vi "GenServer.vi"(8 "error in":errorcluster, 10 "Default Server":T1, 11 "Server":T1) -> (0 "error out":errorcluster, 2 "Unique Handlers":bool, 3 "Lines":string[](array[string]))   [LabVIEW 2017]
uses:
  <vilib>/WebServerConfig/Server.ctl
  <vilib>/WebServerConfig/Alias.ctl
  <vilib>/WebServerConfig/ErrorDocument.ctl
  <vilib>/WebServerConfig/Action.ctl
  <vilib>/WebServerConfig/Redirect.ctl
  <vilib>/WebServerConfig/Interface.ctl
  <vilib>/WebServerConfig/AddHandler.ctl
  <vilib>/WebServerConfig/SSL.ctl
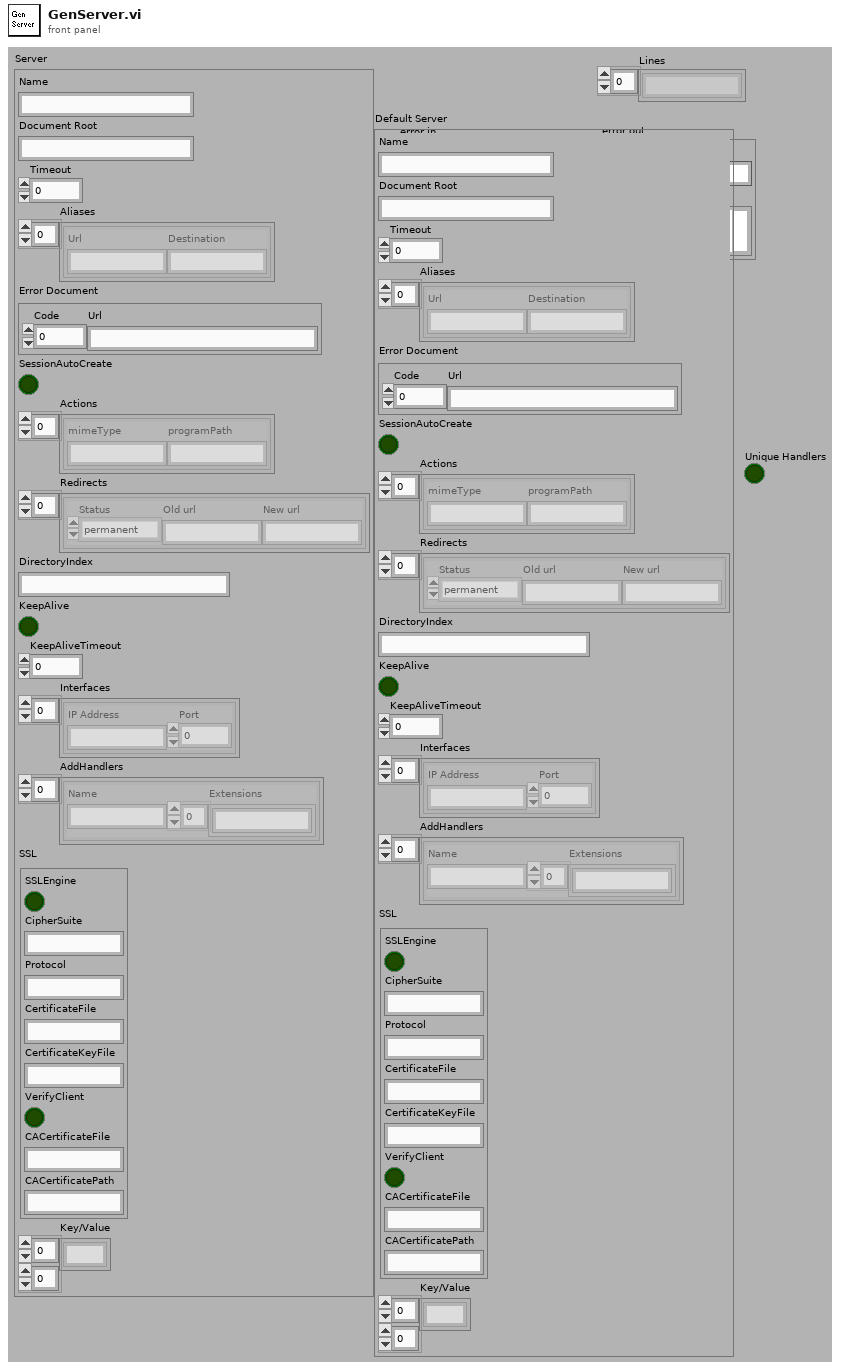
[diagram p1: front panel]
types:
  T1 = typedef "Server.ctl" = cluster{"Name":string, "Document Root":string, "Timeout":u32, "Aliases":T2[], "Error Document":T3, "SessionAutoCreate":bool, "Actions":T4[], "Redirects":T5[], "DirectoryIndex":string, "KeepAlive":bool, "KeepAliveTimeout":u32, "Interfaces":T6[], "AddHandlers":T7[], "SSL":T8, "Key/Value":string[][]}
  T2 = typedef "Alias.ctl" = cluster{"Url":string, "Destination":string}
  T3 = typedef "ErrorDocument.ctl" = cluster{"Code":u16, "Url":string}
  T4 = typedef "Action.ctl" = cluster{"mimeType":string, "programPath":string}
  T5 = typedef "Redirect.ctl" = cluster{"Status":enum16{"permanent", "temp", "seeother", "gone"}, "Old url":string, "New url":string}
  T6 = typedef "Interface.ctl" = cluster{"IP Address":string, "Port":u16}
  T7 = typedef "AddHandler.ctl" = cluster{"Name":string, "Extensions":string[]}
  T8 = typedef "SSL.ctl" = cluster{"SSLEngine":bool, "CipherSuite":string, "Protocol":string, "CertificateFile":string, "CertificateKeyFile":string, "VerifyClient":bool, "CACertificateFile":string, "CACertificatePath":string}
  T9 = enum16{"ServerName", "DocumentRoot", "InactivityTimeout", "AddPipeline", "DirectoryIndex", "Aliases", "ErrorDocument", "SSLEngine", "SSLCertificateFile", "SSLCertificateKeyFile", "SSLVerifyClient", "Key/Value"}
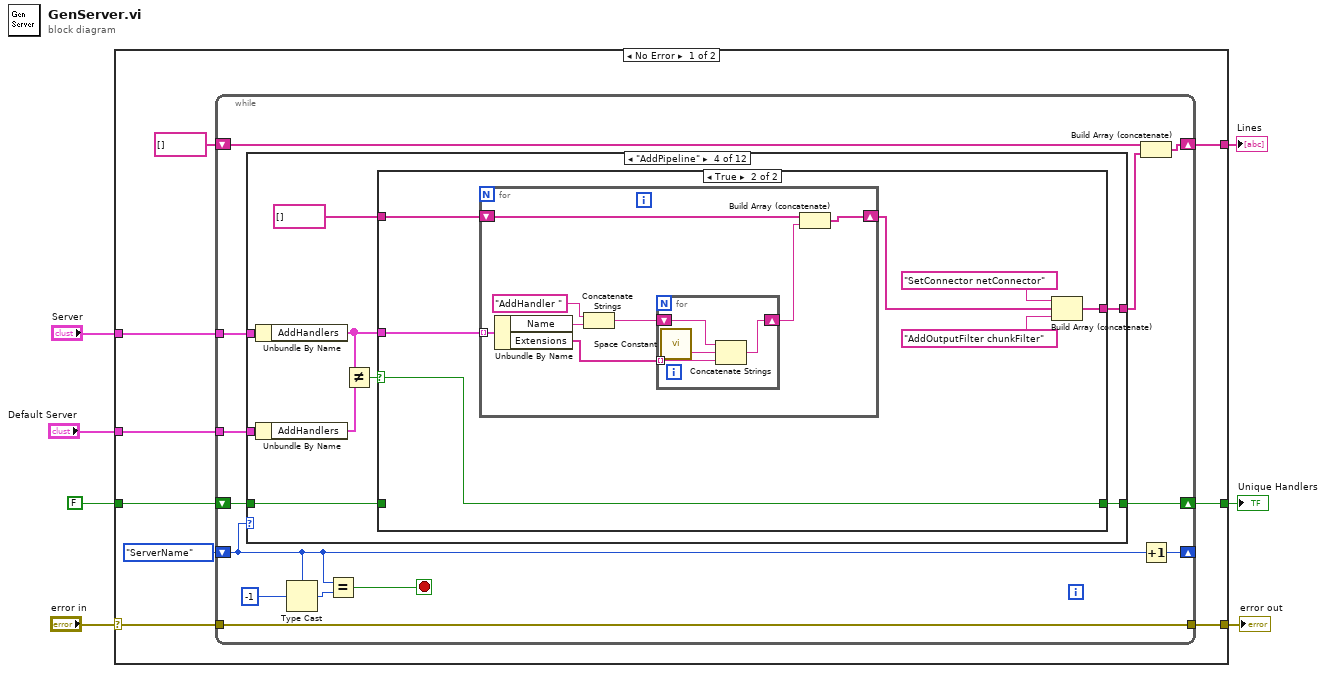
[diagram p0: block diagram]
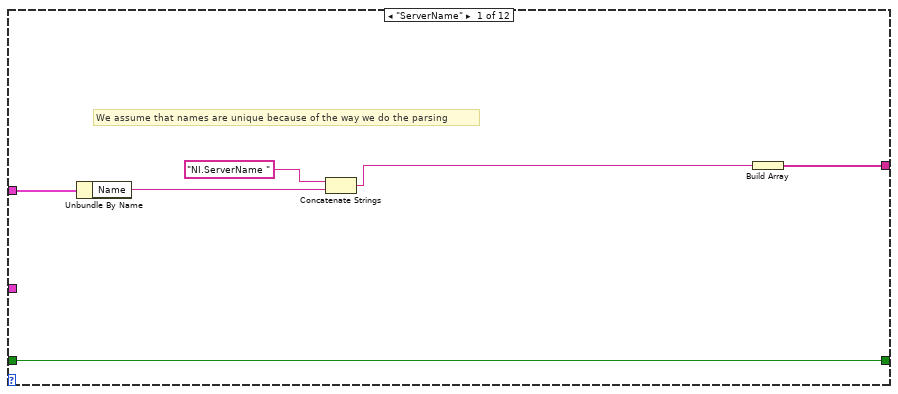
[diagram p2: hidden frame]
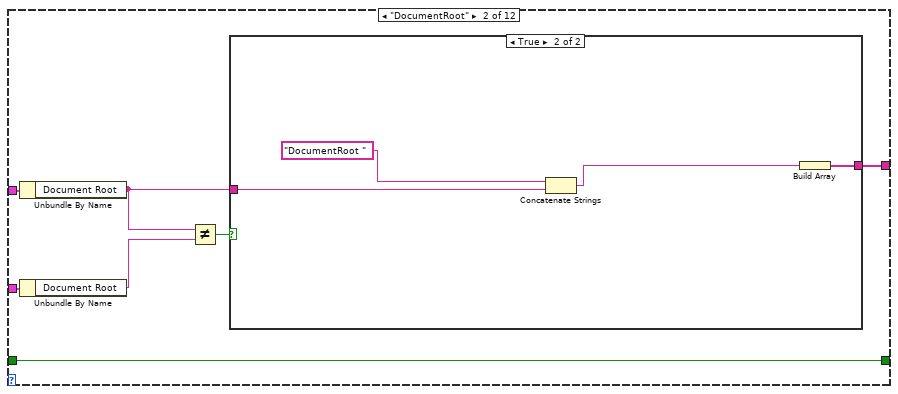
[diagram p3: hidden frame]
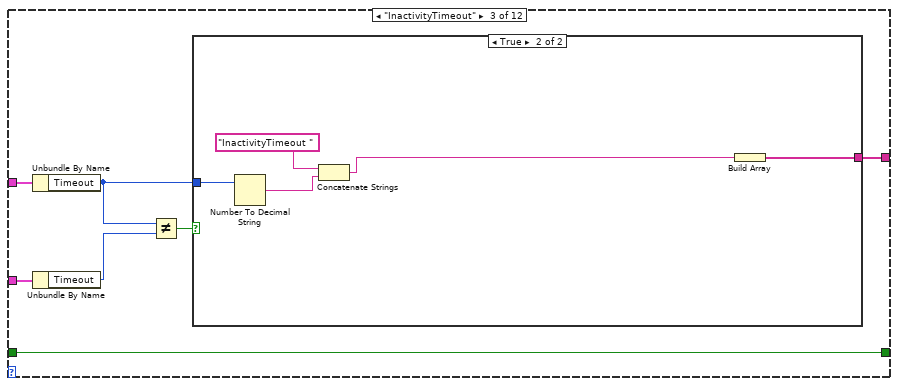
[diagram p5: hidden frame]
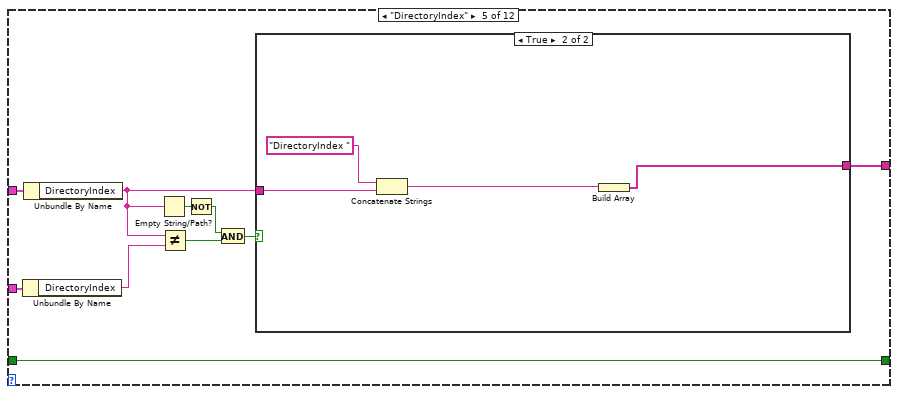
[diagram p8: hidden frame]
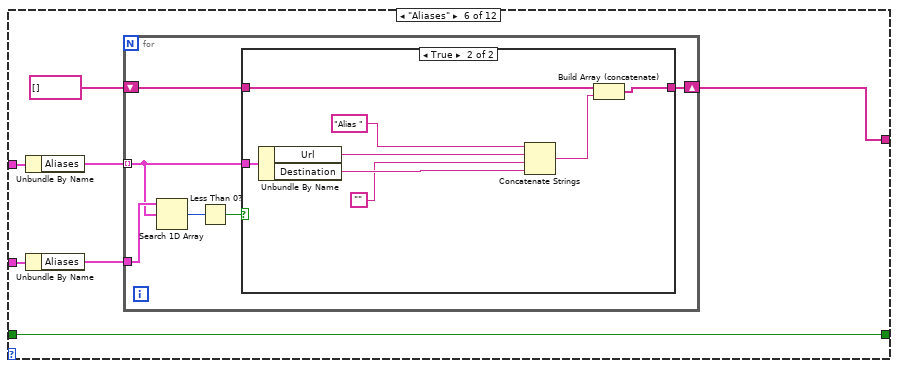
[diagram p10: hidden frame]
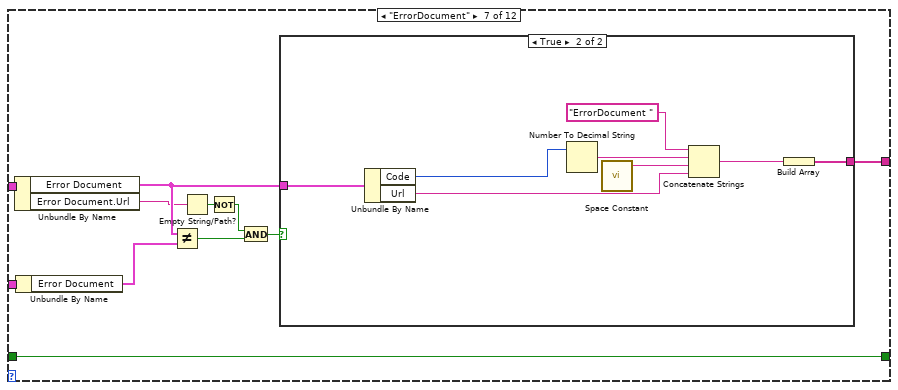
[diagram p12: hidden frame]
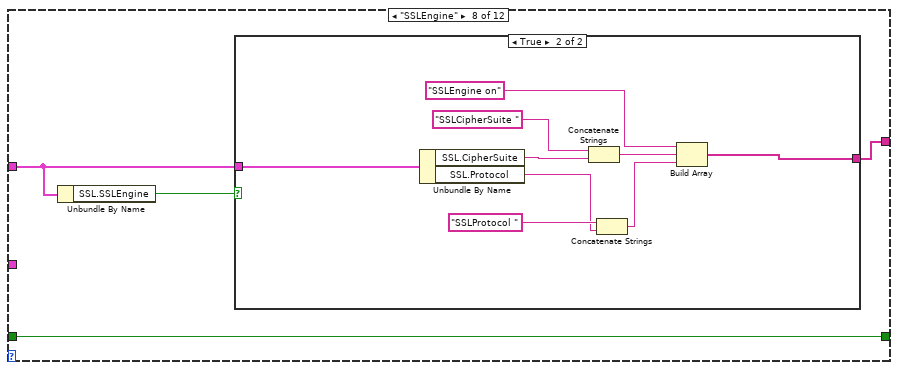
[diagram p14: hidden frame]
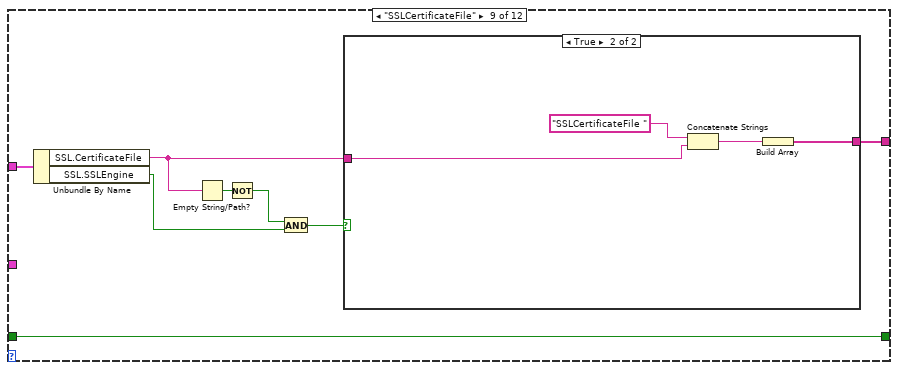
[diagram p16: hidden frame]
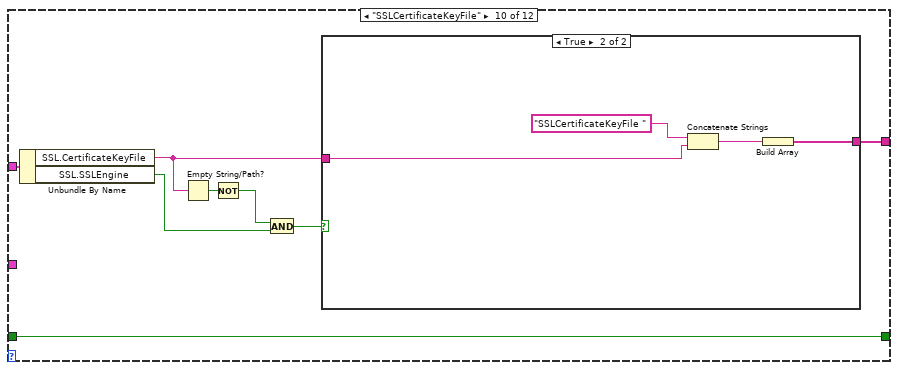
[diagram p18: hidden frame]
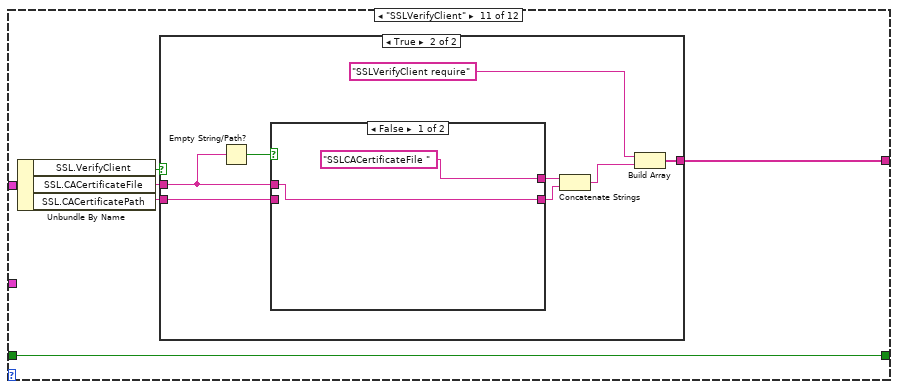
[diagram p20: hidden frame]
diagram:
  n1 = case shown="No Error" "error in" {
    selector: "error in" -> [w13 w209]
    tunnel: [w12 w209] -> w5
    tunnel: "Server" -> [w11 _]
    tunnel: [w16 string[] []] -> w7
    tunnel: "Default Server" -> [w10 _]
    tunnel: [w9 w208] -> w2
    tunnel: FALSE -> [w8 w208]
    frame No Error {
      n2 = while {
        tunnel: w13 -> [w20]
        tunnel: [w20] -> w12
        shift-right: [w26] -> _
        shift-left: T9."ServerName" -> [w25]
        tunnel: w11 -> [w24]
        shift-right: [w22] -> w16
        shift-left: string[] [] -> [w23]
        tunnel: w10 -> [w19]
        shift-right: [w18] -> w9
        shift-left: w8 -> [w17]
        stop <- w27 stop-if-true
        n3 = case shown="\"AddPipeline\"" w25 {
          tunnel: w24 -> [w35 w42 w53 w67 w98 w109 w135 w145 w164 w176 w186 w201]
          tunnel: [w31 w37 w48 w65 w90 w104 w131 w146 w162 w174 w184 w199] -> w21
          tunnel: w19 -> [_ w41 w52 w64 w97 w108 w134 _ _ _ _ _]
          tunnel: [w30 w36 w47 w60 w89 w103 w125 w147 w163 w175 w185 w202] -> w18
          tunnel: w17 -> [w30 w36 w47 w59 w89 w103 w125 w147 w163 w175 w185 w202]
          frame "ServerName" {
            # "We assume that names are unique because of the way we do the parsing"
            n4 = Unbundle By Name(w35) -> ("Name"=w33:string)
            n5 = Concatenate Strings("NI.ServerName " ("string"), w33) -> (w32:string)
            n6 = Build Array(w32) -> (w31:string[])
          }
          frame "DocumentRoot" {
            n7 = Unbundle By Name(w42) -> ("Document Root"=w38:string)
            n8 = Unbundle By Name(w41) -> ("Document Root"=w40:string)
            n9 = Not Equal?(x=w38, y=w40) -> (x != y?=w39:bool)
            n10 = case shown="True" w39 {
              tunnel: w38 -> [_ w44]
              tunnel: [_ w43] -> w37
              frame False {
              }
              frame True {
                n11 = Concatenate Strings("DocumentRoot " ("string"), w44) -> (w46:string)
                n12 = Build Array(w46) -> (w43:string[])
              }
            }
          }
          frame "InactivityTimeout" {
            n13 = Unbundle By Name(w53) -> ("Timeout"=w49:u32)
            n14 = Unbundle By Name(w52) -> ("Timeout"=w51:u32)
            n15 = Not Equal?(x=w49, y=w51) -> (x != y?=w50:bool)
            n16 = case shown="True" w50 {
              tunnel: w49 -> [_ w58]
              tunnel: [_ w54] -> w48
              frame False {
              }
              frame True {
                n17 = Number To Decimal String(number=w58) -> (decimal integer string=w56:string)  [unwired: 1 in]
                n18 = Concatenate Strings("InactivityTimeout " ("string"), w56) -> (w55:string)
                n19 = Build Array(w55) -> (w54:string[])
              }
            }
          }
          frame "AddPipeline" {
            n20 = Unbundle By Name(w67) -> ("AddHandlers"=w63:T7[])
            n21 = Unbundle By Name(w64) -> ("AddHandlers"=w61:T7[])
            n22 = Not Equal?(x=w63, y=w61) -> (x != y?=w62:bool)
            n23 = case shown="True" w62 {
              selector: w62 -> [_ w74]
              tunnel: w63 -> [_ w75]
              tunnel: string[] [] -> [w69 w76]
              tunnel: [w69 w72] -> w65
              tunnel: [w68 w74] -> w60
              tunnel: w59 -> [w68 _]
              frame False {
              }
              frame True {
                n24 = for {
                  tunnel: w75 -> [w82] mode=indexing
                  shift-right: [w84] -> w73
                  shift-left: w76 -> [w83]
                  n25 = Unbundle By Name(w82) -> ("Name"=w79:string, "Extensions"=w81:string[])
                  n26 = Concatenate Strings("AddHandler " ("string"), w79) -> (w77:string)
                  n27 = for {
                    tunnel: w81 -> [w88] mode=indexing
                    shift-right: [w87] -> w80
                    shift-left: w77 -> [w85]
                    n28 = call <vilib>:"Space Constant.vi"() -> ("String"=w86:string)
                    n29 = Concatenate Strings(w85, w86, w88) -> (w87:string)
                  }
                  n30 = Build Array (concatenate)(w83, w80) -> (w84:string[])
                }
                n31 = Build Array (concatenate)("SetConnector netConnector" ("string"), w73, "AddOutputFilter chunkFilter" ("string")) -> (w72:string[])
              }
            }
          }
          frame "DirectoryIndex" {
            n32 = Unbundle By Name(w97) -> ("DirectoryIndex"=w96:string)
            n33 = Unbundle By Name(w98) -> ("DirectoryIndex"=w91:string)
            n34 = Empty String/Path?(string/path=w91) -> (empty?=w93:bool)
            n35 = Not Equal?(x=w91, y=w96) -> (x != y?=w95:bool)
            n36 = Not(x=w93) -> (.not. x?=w92:bool)
            n37 = And(x=w92, y=w95) -> (x .and. y?=w94:bool)
            n38 = case shown="True" w94 {
              tunnel: w91 -> [_ w102]
              tunnel: [_ w99] -> w90
              frame False {
              }
              frame True {
                n39 = Concatenate Strings("DirectoryIndex " ("string"), w102) -> (w100:string)
                n40 = Build Array(w100) -> (w99:string[])
              }
            }
          }
          frame "Aliases" {
            n41 = Unbundle By Name(w109) -> ("Aliases"=w107:T2[])
            n42 = Unbundle By Name(w108) -> ("Aliases"=w106:T2[])
            n43 = for {
              tunnel: w107 -> [w112] mode=indexing
              tunnel: w106 -> [w115]
              shift-right: [w110] -> w104
              shift-left: string[] [] -> [w111]
              n44 = Search 1D Array(1D array=w115, element=w112) -> (index of element=w114:i32)  [unwired: 1 in]
              n45 = Less Than 0?(x=w114) -> (x < 0?=w113:bool)
              n46 = case shown="True" w113 {
                tunnel: w112 -> [_ w124]
                tunnel: w111 -> [w116 w117]
                tunnel: [w116 w118] -> w110
                frame False {
                }
                frame True {
                  n47 = Unbundle By Name(w124) -> ("Url"=w122:string, "Destination"=w123:string)
                  n48 = Concatenate Strings("Alias " ("string"), w122, "", w123) -> (w119:string)
                  n49 = Build Array (concatenate)(w117, w119) -> (w118:string[])
                }
              }
            }
          }
          frame "ErrorDocument" {
            n50 = Unbundle By Name(w135) -> ("Error Document"=w132:T3, "Error Document.Url"=w126:string)
            n51 = Unbundle By Name(w134) -> ("Error Document"=w133:T3)
            n52 = Not Equal?(x=w132, y=w133) -> (x != y?=w127:bool)
            n53 = Empty String/Path?(string/path=w126) -> (empty?=w130:bool)
            n54 = Not(x=w130) -> (.not. x?=w129:bool)
            n55 = And(x=w129, y=w127) -> (x .and. y?=w128:bool)
            n56 = case shown="True" w128 {
              tunnel: w132 -> [_ w143]
              tunnel: [_ w136] -> w131
              frame False {
              }
              frame True {
                n57 = Unbundle By Name(w143) -> ("Code"=w142:u16, "Url"=w138:string)
                n58 = Number To Decimal String(number=w142) -> (decimal integer string=w140:string)  [unwired: 1 in]
                n59 = call <vilib>:"Space Constant.vi"() -> ("String"=w139:string)
                n60 = Concatenate Strings("ErrorDocument " ("string"), w140, w139, w138) -> (w137:string)
                n61 = Build Array(w137) -> (w136:string[])
              }
            }
          }
          frame "SSLEngine" {
            n62 = Unbundle By Name(w145) -> ("SSL.SSLEngine"=w144:bool)
            n63 = case shown="True" w144 {
              tunnel: [_ w156] -> w146
              tunnel: w145 -> [_ w155]
              frame False {
              }
              frame True {
                n64 = Unbundle By Name(w155) -> ("SSL.CipherSuite"=w152:string, "SSL.Protocol"=w151:string)
                n65 = Concatenate Strings("SSLCipherSuite " ("string"), w152) -> (w149:string)
                n66 = Concatenate Strings("SSLProtocol " ("string"), w151) -> (w150:string)
                n67 = Build Array("SSLEngine on" ("string"), w149, w150) -> (w156:string[])
              }
            }
          }
          frame "SSLCertificateFile" {
            n68 = Unbundle By Name(w164) -> ("SSL.CertificateFile"=w160:string, "SSL.SSLEngine"=w159:bool)
            n69 = Empty String/Path?(string/path=w160) -> (empty?=w161:bool)
            n70 = Not(x=w161) -> (.not. x?=w158:bool)
            n71 = And(x=w158, y=w159) -> (x .and. y?=w157:bool)
            n72 = case shown="True" w157 {
              tunnel: w160 -> [_ w165]
              tunnel: [_ w168] -> w162
              frame False {
              }
              frame True {
                n73 = Concatenate Strings("SSLCertificateFile " ("string"), w165) -> (w167:string)
                n74 = Build Array(w167) -> (w168:string[])
              }
            }
          }
          frame "SSLCertificateKeyFile" {
            n75 = Unbundle By Name(w176) -> ("SSL.CertificateKeyFile"=w172:string, "SSL.SSLEngine"=w171:bool)
            n76 = Empty String/Path?(string/path=w172) -> (empty?=w173:bool)
            n77 = Not(x=w173) -> (.not. x?=w170:bool)
            n78 = And(x=w170, y=w171) -> (x .and. y?=w169:bool)
            n79 = case shown="True" w169 {
              tunnel: w172 -> [_ w177]
              tunnel: [_ w180] -> w174
              frame False {
              }
              frame True {
                n80 = Concatenate Strings("SSLCertificateKeyFile " ("string"), w177) -> (w179:string)
                n81 = Build Array(w179) -> (w180:string[])
              }
            }
          }
          frame "SSLVerifyClient" {
            n82 = Unbundle By Name(w186) -> ("SSL.VerifyClient"=w183:bool, "SSL.CACertificateFile"=w182:string, "SSL.CACertificatePath"=w181:string)
            n83 = case shown="True" w183 {
              tunnel: [_ w194] -> w184
              tunnel: w182 -> [_ w191]
              tunnel: w181 -> [_ w190]
              frame False {
              }
              frame True {
                n84 = Empty String/Path?(string/path=w191) -> (empty?=w192:bool)
                n85 = case shown="False" w192 {
                  tunnel: w191 -> [w195 _]
                  tunnel: w190 -> [_ w197]
                  tunnel: ["SSLCACertificateFile " ("string") "SSLCACertificatePath " ("string")] -> w189
                  tunnel: [w195 w197] -> w188
                  frame False {
                  }
                  frame True {
                  }
                }
                n86 = Concatenate Strings(w189, w188) -> (w187:string)
                n87 = Build Array("SSLVerifyClient require" ("string"), w187) -> (w194:string[])
              }
            }
          }
          frame "Key/Value" {
            n88 = Unbundle By Name(w201) -> ("Key/Value"=w200:string[][])
            n89 = for {
              tunnel: w200 -> [w206] mode=indexing
              tunnel: [w203] -> w199 mode=indexing
              n90 = Index Array(array=w206) -> (element #1=w205:string, element #2=w204:string)  [unwired: 2 in]
              n91 = call <vilib>:"Space Constant.vi"() -> ("String"=w207:string)
              n92 = Concatenate Strings(w205, w207, w204) -> (w203:string)
            }
          }
        }
        n93 = Type Cast(type=w25, x=-1) -> (*(type *) &x=w28:T9)
        n94 = Equal?(x=w25, y=w28) -> (x = y?=w27:bool)
        n95 = Build Array (concatenate)(w23, w21) -> (w22:string[])
        n96 = Increment(x=w25) -> (x+1=w26:T9)
      }
    }
    frame Error {
    }
  }
  "Lines" <- w7
  "error out" <- w5
  "Unique Handlers" <- w2
